vi "Stage_Controller.vi"(2 "Error In":errorcluster, 3 "Mirror Switch":bool) -> (0 "Error Out":errorcluster, 1 "Indicator":bool=TRUE)   [LabVIEW 2013]
uses:
  <vilib>/Utility/miscctls.llb/LVPointTypeDef.ctl
  <vilib>/DAQmx/write.llb/DAQmx Write (Digital Bool 1Line 1Point).vi
  <vilib>/Utility/config.llb/Read Key (Boolean).vi
  <vilib>/Utility/config.llb/Write Key (Boolean).vi
  <vilib>/Instr/_visa.llb/VISA Configure Serial Port (Instr).vi
  <vilib>/DAQmx/create/channels.llb/DAQmx Create Channel (DO-Digital Output).vi
  <vilib>/DAQmx/miscellaneous.llb/DAQmx Fill In Error Info.vi
  <vilib>/Utility/config.llb/NI_LVConfig.lvlib
panel:
  out "number":i32
  in  "Resource Name":refnum<visa-resource-name>="COM3"
  out "Slide":u8(slide) scale=0.0..100.0
  in  "stop":bool
  in  "Stop Button":bool caption="stop"
  # "CCLDAS Mirror Stepper Motor Control V4.000"
  # "Mirror Out"
  # "Mirror In"
  # "Optimal position is when the right side of the slot is on 43 mm and the dial is at ~ 3.2."
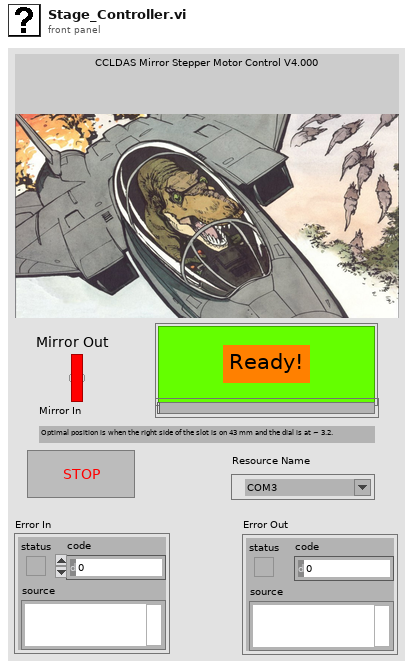
[diagram p1: front panel]
types:
  T1 = typedef "LVPointTypeDef.ctl" = cluster{"Horizontal":i16, "Vertical":i16}
  T2 = typedef "NI_LVConfig.lvlib/Config Data RefNum.ctl" = refnum<k1>
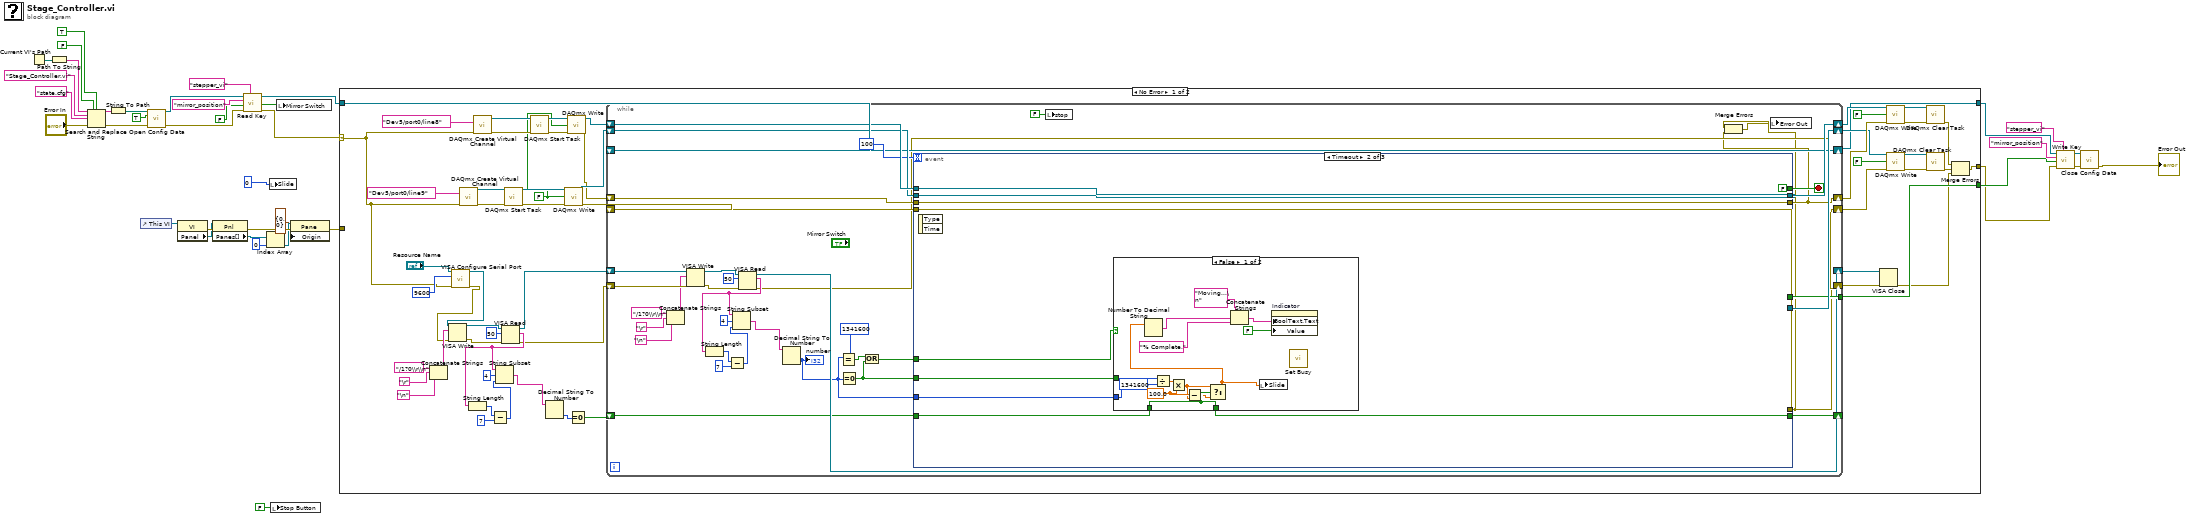
[diagram p0: block diagram]
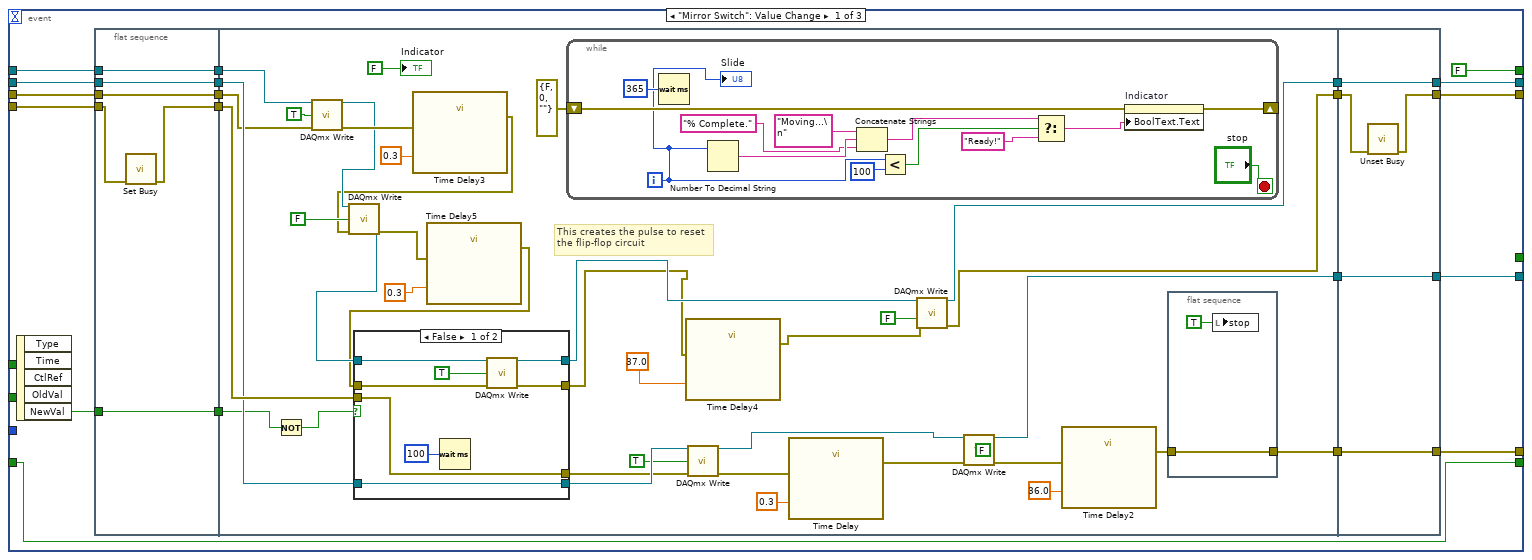
[diagram p2: hidden frame]
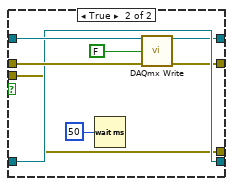
[diagram p3: hidden frame]
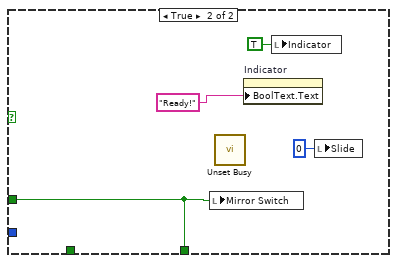
[diagram p4: hidden frame]
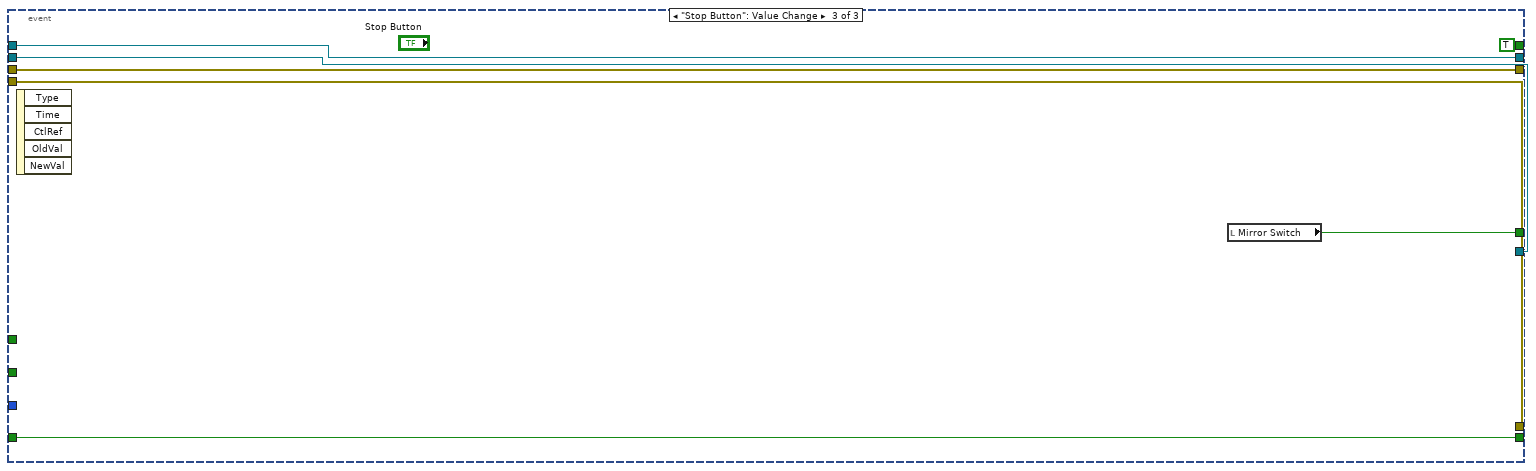
[diagram p5: hidden frame]
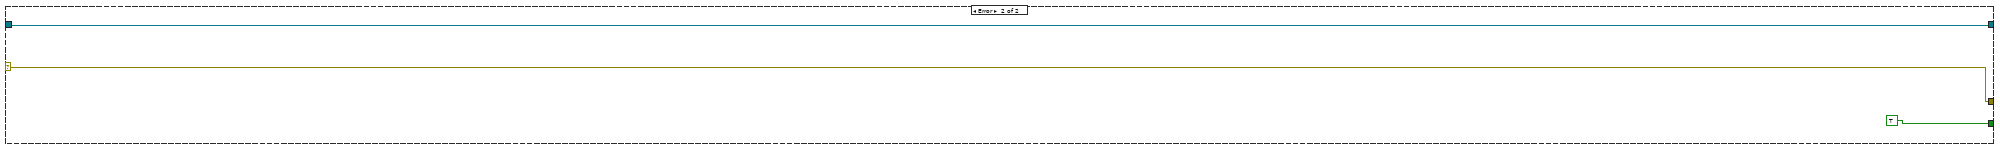
[diagram p6: hidden frame]
diagram:
  n1 = Current VI's Path() -> (path=w23:path)
  n2 = Path To String(path=w23) -> (string=w21:string)
  n3 = Search and Replace String(replace all?=FALSE ("ignore case? (F)"), case sensitive?=TRUE ("ignore case? (F)"), input string=w21, search string="Stage_Controller.vi" ("section"), replace string="state.cfg" ("string"), error in="Error In") -> (result string=w16:string, error out=w14:errorcluster)  [unwired: 2 in, 2 out]
  n4 = String To Path(string=w16) -> (path=w22:path)
  n5 = control-ref of="This VI"() -> (w9:refnum<vi>)
  n6 = call <vilib>:"Open Config Data.vi"("error in (no error)"=w14, "create file if necessary (T)"=TRUE, "configuration file path"=w22) -> ("error out"=w35:errorcluster, "refnum"=w36:T2)  [unwired: 6 in, 1 out]
  n7 = property class="VI"(reference=w9) -> (error out=w8:errorcluster, "Panel"=w7:refnum<vi>)  [unwired: 1 in, 1 out]
  n8 = property class="Pnl"(reference=w7, error in=w8) -> (error out=w6:errorcluster, "Panes[]"=w5:refnum<vi>[])  [unwired: 1 out]
  n9 = call-poly <vilib>:"Read Key.vi"("section"="stepper_vi", "error in (no error)"=w35, "default value"=FALSE, "key"="mirror_position" ("section"), "refnum"=w36) -> ("error out"=w25:errorcluster, "value"=w37:bool, "refnum out"=w34:T2)  [unwired: 3 in, 1 out]
  n10 = Index Array(array=w5, index=0) -> (element=w3:refnum<vi>)
  n11 = local write "Slide"(u8 0 ("Slide")) -> ()
  n12 = local write "Stop Button"(FALSE ("Stop Button")) -> ()
  n13 = local write "Mirror Switch"(w37) -> ()
  n14 = property class="Pane"(reference=w3, error in=w6, "Origin"=T1 {"Horizontal"=0, "Vertical"=0}) -> (error out=w2:errorcluster)  [unwired: 1 out]
  n15 = case shown="No Error" w25 {
    selector: w25 -> [w66 w269]
    tunnel: [w73 w269] -> w10
    tunnel: w34 -> [w71 w268]
    tunnel: [w70 w268] -> w33
    tunnel: [w69 TRUE] -> w12
    tunnel: w2 -> [_ _]
    frame No Error {
      w58 = FALSE ("data")
      n16 = Concatenate Strings("/1?0\\r\\n" ("string"), "\r", "\n") -> (w55:string)
      n17 = call-poly "VISA Configure Serial Port"("VISA resource name"="Resource Name", "baud rate (9600)"=9600, "error in (no error)"=w66) -> ("VISA resource name out"=w44:refnum<visa-resource-name>, "error out"=w43:errorcluster)  [unwired: 11 in]
      n18 = VISA Write(VISA resource name=w44, write buffer=w55, error in (no error)=w43) -> (VISA resource name out=w52:refnum<visa-resource-name>, error out=w51:errorcluster)  [unwired: 1 out]
      n19 = call-poly <vilib>:"DAQmx Create Virtual Channel.vi"("lines"=tag "Dev5/port0/line9" ("Button Channel"), "error in"=w66) -> ("task out"=w92:refnum<k21>, "error out"=w91:errorcluster)  [unwired: 12 in]
      n20 = call-poly <vilib>:"DAQmx Create Virtual Channel.vi"("lines"=tag "Dev5/port0/line8" ("Switch Channel"), "error in"=w66) -> ("task out"=w94:refnum<k21>, "error out"=w93:errorcluster)  [unwired: 12 in]
      n21 = VISA Read(VISA resource name=w52, byte count=u32 50, error in (no error)=w51) -> (VISA resource name out=w42:refnum<visa-resource-name>, read buffer=w46:string, error out=w41:errorcluster)  [unwired: 1 out]
      n22 = String Length(string=w46) -> (length=w49:i32)
      n23 = Subtract(x=w49, y=7) -> (x-y=w48:i32)
      n24 = String Subset(string=w46, offset (0)=4, length (rest)=w48) -> (substring=w45:string)
      n25 = call <vilib>:"DAQmx Start Task.vi"("task/channels in"=w92, "error in"=w91) -> ("task out"=w76:refnum<k21>, "error out"=w75:errorcluster)  [unwired: 12 in]
      n26 = call <vilib>:"DAQmx Start Task.vi"("task/channels in"=w94, "error in"=w93) -> ("task out"=w60:refnum<k21>, "error out"=w59:errorcluster)  [unwired: 12 in]
      n27 = Decimal String To Number(string=w45) -> (number=w40:i32)  [unwired: 2 in, 1 out]
      n28 = call-poly <vilib>:"DAQmx Write.vi"("task/channels in"=w76, "data"=w58, "error in"=w75) -> ("task out"=w74:refnum<k21>, "error out"=w72:errorcluster)  [unwired: 10 in, 1 out]
      n29 = call-poly <vilib>:"DAQmx Write.vi"("task/channels in"=w60, "data"=w58, "error in"=w59) -> ("task out"=w62:refnum<k21>, "error out"=w61:errorcluster)  [unwired: 10 in, 1 out]
      n30 = Equal To 0?(x=w40) -> (x = 0?=w39:bool)
      n31 = while {
        shift-right: [w99] -> w86
        shift-left: w61 -> [w131]
        shift-right: [w98] -> w80
        shift-left: w72 -> [w129]
        shift-right: [w123] -> w70
        shift-left: w71 -> [w123]
        tunnel: [w122] -> w69
        shift-right: [w128] -> w85
        shift-left: w62 -> [w132]
        shift-right: [w127] -> w81
        shift-left: w74 -> [w130]
        shift-right: [w95] -> _
        shift-left: w39 -> [w96]
        shift-right: [w107] -> w65
        shift-left: w42 -> [w121]
        shift-right: [w106] -> w64
        shift-left: w41 -> [w120]
        stop <- w126 stop-if-true
        n32 = Concatenate Strings("/1?0\\r\\n" ("string"), "\r", "\n") -> (w117:string)
        n33 = VISA Write(VISA resource name=w121, write buffer=w117, error in (no error)=w120) -> (VISA resource name out=w114:refnum<visa-resource-name>, error out=w113:errorcluster)  [unwired: 1 out]
        n34 = VISA Read(VISA resource name=w114, byte count=u32 50, error in (no error)=w113) -> (VISA resource name out=w107:refnum<visa-resource-name>, read buffer=w108:string, error out=w106:errorcluster)  [unwired: 1 out]
        n35 = String Length(string=w108) -> (length=w111:i32)
        n36 = Subtract(x=w111, y=7) -> (x-y=w110:i32)
        n37 = String Subset(string=w108, offset (0)=4, length (rest)=w110) -> (substring=w105:string)
        n38 = Decimal String To Number(string=w105) -> (number=w100:i32)  [unwired: 2 in, 1 out]
        "number" <- w100
        n39 = Equal?(x=w100, y=1341600) -> (x = y?=w103:bool)
        n40 = Equal To 0?(x=w100) -> (x = 0?=w101:bool)
        n41 = Or(x=w103, y=w101) -> (x .or. y?=w102:bool)
        n42 = event shown="[1] Timeout" {
          selector: _ -> [_ _ _]
          dyn-events: _ -> [_ _ _]
          timeout: 100 -> [_ _ _]
          tunnel: w132 -> [w146 w241 w266]
          tunnel: w131 -> [w144 w242 w265]
          tunnel: w130 -> [w147 w239 w264]
          tunnel: w129 -> [w150 w240 w263]
          tunnel: [w149 w241 w266] -> w128
          tunnel: [w148 w242 w265] -> w99
          tunnel: [w152 w239 w264] -> w127
          tunnel: [w143 w240 w263] -> w98
          tunnel: [FALSE ("Stop Button") FALSE ("Stop Button") TRUE ("Stop Button")] -> w126
          tunnel: [_ _ w261] -> w122
          tunnel: w102 -> [_ w237 _]
          tunnel: w101 -> [_ w236 _]
          tunnel: w100 -> [_ w235 _]
          tunnel: w96 -> [w133 w234 w260]
          tunnel: [w133 w233 w260] -> w95
          event "Mirror Switch": Value Change {
            n43 = event-data() -> ("NewVal"=w145:bool)  [unwired: 1 in, 4 out]
            n44 = flat-sequence {
              tunnel: w144 -> [w155]
              tunnel: w145 -> [w156]
              tunnel: w146 -> [w157]
              tunnel: w147 -> [w158]
              tunnel: w150 -> [w154]
              tunnel: [w153] -> w142
              tunnel: [w158] -> w141
              tunnel: [w157] -> w140
              tunnel: [w156] -> w139
              tunnel: [w155] -> w138
              tunnel: w142 -> [w183]
              tunnel: w141 -> [w169]
              tunnel: w140 -> [w167]
              tunnel: w139 -> [w163]
              tunnel: w138 -> [w161]
              tunnel: [w191] -> w137
              tunnel: [w173] -> w136
              tunnel: [w170] -> w135
              tunnel: [w159] -> w134
              tunnel: [w230] -> w143
              tunnel: [w228] -> w148
              tunnel: [w231] -> w149
              tunnel: [w232] -> w152
              tunnel: w137 -> [w232]
              tunnel: w136 -> [w231]
              tunnel: w135 -> [w229]
              tunnel: w134 -> [w230]
              frame #0 {
                n45 = call <vilib>:"Set Busy.vi"("error in (no error)"=w154) -> ("error out"=w153:errorcluster)  [unwired: 9 in, 1 out]
              }
              frame #1 {
                # "This creates the pulse to reset\nthe flip-flop circuit"
                n46 = Not(x=w163) -> (.not. x?=w162:bool)
                n47 = call-poly <vilib>:"DAQmx Write.vi"("task/channels in"=w167, "data"=TRUE, "error in"=w161) -> ("task out"=w178:refnum<k21>, "error out"=w181:errorcluster)  [unwired: 10 in, 1 out]
                n48 = call "Time Delay3"("error in (no error)"=w181, "Delay Time (s)"=0.3) -> ("error out"=w177:errorcluster)  [unwired: 9 in]
                n49 = call-poly <vilib>:"DAQmx Write.vi"("task/channels in"=w178, "data"=FALSE, "error in"=w177) -> ("task out"=w168:refnum<k21>, "error out"=w166:errorcluster)  [unwired: 10 in, 1 out]
                n50 = call "Time Delay5"("error in (no error)"=w166, "Delay Time (s)"=0.3) -> ("error out"=w165:errorcluster)  [unwired: 9 in]
                n51 = case shown="False" w162 {
                  tunnel: w168 -> [w217 w227]
                  tunnel: w165 -> [w216 w226]
                  tunnel: w169 -> [w219 w224]
                  tunnel: w183 -> [w218 w223]
                  tunnel: [w219 w224] -> w196
                  tunnel: [w218 w223] -> w195
                  tunnel: [w214 w222] -> w174
                  tunnel: [w213 w221] -> w171
                  frame False {
                    n52 = Wait (ms)(milliseconds to wait=u32 100) -> ()  [unwired: 1 out]
                    n53 = call-poly <vilib>:"DAQmx Write.vi"("task/channels in"=w217, "data"=TRUE, "error in"=w216) -> ("task out"=w214:refnum<k21>, "error out"=w213:errorcluster)  [unwired: 10 in, 1 out]
                  }
                  frame True {
                    n54 = Wait (ms)(milliseconds to wait=u32 50) -> ()  [unwired: 1 out]
                    n55 = call-poly <vilib>:"DAQmx Write.vi"("task/channels in"=w227, "data"=FALSE, "error in"=w226) -> ("task out"=w222:refnum<k21>, "error out"=w221:errorcluster)  [unwired: 10 in, 1 out]
                  }
                }
                n56 = while {
                  shift-right: [w201] -> _
                  shift-left: errorcluster {"status"=FALSE, "code"=0, "source"=""} ("error out") -> [w200]
                  i -> [w199]
                  stop <- "stop" stop-if-true
                  n57 = Wait (ms)(milliseconds to wait=u32 365) -> ()  [unwired: 1 out]
                  n58 = Number To Decimal String(number=w199) -> (decimal integer string=w209:string)  [unwired: 1 in]
                  n59 = Concatenate Strings("Moving...\n" ("string"), w209, "% Complete." ("string")) -> (w205:string)
                  n60 = Less?(x=w199, y=100) -> (x < y?=w204:bool)
                  n61 = Select(t=w205, s=w204, f="Ready!") -> (s? t:f=w202:string)
                  n62 = property on="Indicator" class="Bool (strict)"(error in=w200, "BoolText.Text"=w202) -> (error out=w201:errorcluster)  [unwired: 1 in, 1 out]
                  "Slide" <- w199
                }
                n63 = call "Time Delay4"("error in (no error)"=w171, "Delay Time (s)"=37.0) -> ("error out"=w172:errorcluster)  [unwired: 9 in]
                n64 = call-poly <vilib>:"DAQmx Write.vi"("task/channels in"=w196, "data"=TRUE, "error in"=w195) -> ("task out"=w193:refnum<k21>, "error out"=w189:errorcluster)  [unwired: 10 in, 1 out]
                n65 = call "Time Delay"("error in (no error)"=w189, "Delay Time (s)"=0.3) -> ("error out"=w188:errorcluster)  [unwired: 9 in]
                n66 = call-poly <vilib>:"DAQmx Write.vi"("task/channels in"=w174, "data"=FALSE, "error in"=w172) -> ("task out"=w173:refnum<k21>, "error out"=w170:errorcluster)  [unwired: 10 in, 1 out]
                n67 = call-poly <vilib>:"DAQmx Write.vi"("task/channels in"=w193, "data"=FALSE, "error in"=w188) -> ("task out"=w191:refnum<k21>, "error out"=w187:errorcluster)  [unwired: 10 in, 1 out]
                n68 = call "Time Delay2"("error in (no error)"=w187, "Delay Time (s)"=36.0) -> ("error out"=w186:errorcluster)  [unwired: 9 in]
                n69 = flat-sequence {
                  tunnel: w186 -> [w198]
                  tunnel: [w198] -> w159
                  frame #0 {
                    n70 = local write "stop"(TRUE ("stop")) -> ()
                  }
                }
                "Indicator" <- FALSE
              }
              frame #2 {
                n71 = call <vilib>:"Unset Busy.vi"("error in (no error)"=w229) -> ("error out"=w228:errorcluster)  [unwired: 10 in]
              }
            }
          }
          event Timeout {
            n72 = event-data() -> ()  [unwired: 1 in, 2 out]
            n73 = case shown="False" w237 {
              tunnel: w236 -> [_ w256]
              tunnel: w235 -> [w252 _]
              tunnel: w234 -> [w245 _]
              tunnel: [w245 w256] -> w233
              frame False {
                w249 = 100.0 ("y")
                n74 = Divide(x=w252, y=1341600) -> (x/y=w250:dbl)
                n75 = Multiply(x=w250, y=w249) -> (x*y=w243:dbl)
                n76 = Subtract(x=w249, y=w243) -> (x-y=w244:dbl)
                n77 = Select(t=w243, s=w245, f=w244) -> (s? t:f=w246:dbl)
                n78 = Number To Decimal String(number=w246) -> (decimal integer string=w248:string)  [unwired: 1 in]
                n79 = Concatenate Strings("Moving...\n" ("string"), w248, "% Complete." ("string")) -> (w247:string)
                n80 = local write "Slide"(w246) -> ()
                n81 = property on="Indicator" class="Bool (strict)"("BoolText.Text"=w247, "Value"=FALSE ("Indicator")) -> ()  [unwired: 2 in, 2 out]
                n82 = call <vilib>:"Set Busy.vi"() -> ()  [unwired: 10 in, 2 out]
              }
              frame True {
                n83 = local write "Mirror Switch"(w256) -> ()
                n84 = call <vilib>:"Unset Busy.vi"() -> ()  [unwired: 11 in, 1 out]
                n85 = property on="Indicator" class="Bool (strict)"("BoolText.Text"="Ready!" ("f")) -> ()  [unwired: 2 in, 2 out]
                n86 = local write "Indicator"(TRUE ("Indicator")) -> ()
                n87 = local write "Slide"(u8 0 ("Slide")) -> ()
              }
            }
          }
          event "Stop Button": Value Change {
            n88 = event-data() -> ()  [unwired: 1 in, 5 out]
            n89 = local read "Mirror Switch"() -> (w261:bool)
          }
        }
        n90 = local write "stop"(FALSE ("stop")) -> ()
        n91 = Merge Errors(w98, w99) -> (w97:errorcluster)
        n92 = local write "Error Out"(w97) -> ()
      }
      n93 = VISA Close(VISA resource name=w65, error in (no error)=w64) -> (error out=w63:errorcluster)
      n94 = call-poly <vilib>:"DAQmx Write.vi"("task/channels in"=w85, "data"=FALSE, "error in"=w86) -> ("task out"=w84:refnum<k21>, "error out"=w83:errorcluster)  [unwired: 10 in, 1 out]
      n95 = call-poly <vilib>:"DAQmx Write.vi"("task/channels in"=w81, "data"=FALSE, "error in"=w80) -> ("task out"=w79:refnum<k21>, "error out"=w78:errorcluster)  [unwired: 10 in, 1 out]
      n96 = call <vilib>:"DAQmx Clear Task.vi"("task in"=w84, "error in"=w83) -> ("error out"=w90:errorcluster)  [unwired: 13 in]
      n97 = call <vilib>:"DAQmx Clear Task.vi"("task in"=w79, "error in"=w78) -> ("error out"=w89:errorcluster)  [unwired: 13 in]
      n98 = Merge Errors(w90, w89, w63) -> (w73:errorcluster)
    }
    frame Error {
    }
  }
  n99 = call-poly <vilib>:"Write Key.vi"("section"="stepper_vi", "error in (no error)"=w10, "value"=w12, "key"="mirror_position" ("section"), "refnum"=w33) -> ("error out"=w32:errorcluster, "refnum out"=w31:T2)  [unwired: 4 in, 1 out]
  n100 = call <vilib>:"Close Config Data.vi"("error in (no error)"=w32, "refnum"=w31) -> ("error out"=→"Error Out":errorcluster)  [unwired: 8 in, 1 out]
